vi "Read Tektronix WFM.vi"(8 "Error In":errorcluster, 11 "WFM file Path":path) -> (0 "Error Out":errorcluster, 2 "Waveform out":waveform(dbl), 3 "File out":path)   [LabVIEW 2015]
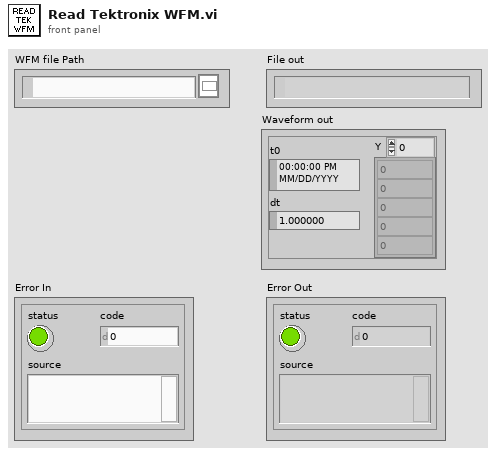
[diagram p1: front panel]
types:
  T1 = typedef "WFM header.ctl" = cluster{"Byte order":u16, "Version":string, "Byte count digits":u8, "Bytes to EOF":i32, "Bytes per point":u8, "Offset of curve buffer":i32, "Label":string, "Number of frames":i32, "Size of header":u16, "Set type":i32, "Number of sets":i32, "Imp dim ref count":i32, "Exp dim ref count":i32, "Data type":i32, "Curve ref count":i32, "Requested FF":i32, "Acquired FF":i32, "Exp dimension 1":T2, "Exp dimension 2":T2, "Imp dimension 1":T3, "Imp dimension 2":T3, "Precharge start offset":i32, "Data start offset":i32, "Postcharge start offset":i32, "Postcharge stop offset":i32, "End of curve buffer offset":i32}
  T2 = typedef "WFM exp dimension.ctl" = cluster{"Scale":dbl, "Offset":dbl, "Size":i32, "Units":string, "Ref point":dbl, "Format":i32, "Storage type":i32, "Trig delay":dbl}
  T3 = typedef "WFM impl dimension.ctl" = cluster{"Scale":dbl, "Offset":dbl, "Size":i32, "Units":string, "Ref point":dbl, "Spacing":i32, "Trig delay":dbl}
  T4 = typedef "WFM file ref.ctl" = cluster{"refnum":refnum<file>, "byte order":enum16{"big-endian, network order", "native, host order", "little-endian"}, "Version":i32}
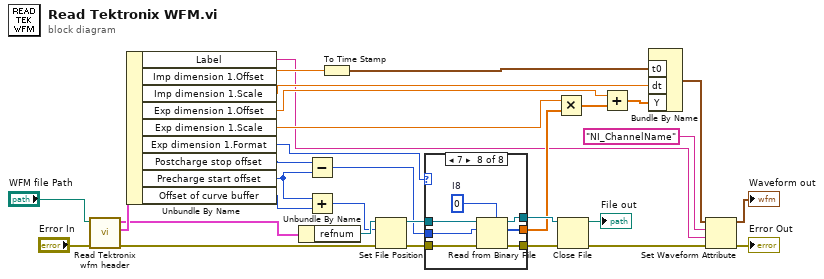
[diagram p0: block diagram]
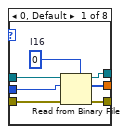
[diagram p2: hidden frame]
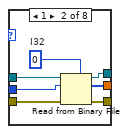
[diagram p3: hidden frame]
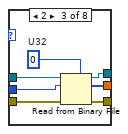
[diagram p4: hidden frame]
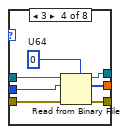
[diagram p5: hidden frame]
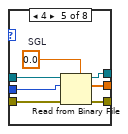
[diagram p6: hidden frame]
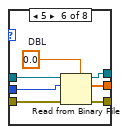
[diagram p7: hidden frame]
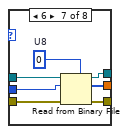
[diagram p8: hidden frame]
diagram:
  n1 = call "Read Tektronix wfm header.vi"("Error In"="Error In", "File Path"="WFM file Path") -> ("Error Out"=w26:errorcluster, "Partial WFM header"=w30:T1, "WFM file ref out"=w29:T4)  [unwired: 7 in]
  n2 = Unbundle By Name(w30) -> ("Label"=w1:string, "Imp dimension 1.Offset"=w18:dbl, "Imp dimension 1.Scale"=w17:dbl, "Exp dimension 1.Offset"=w15:dbl, "Exp dimension 1.Scale"=w14:dbl, "Exp dimension 1.Format"=w12:i32, "Postcharge stop offset"=w11:i32, "Precharge start offset"=w8:i32, "Offset of curve buffer"=w9:i32)
  n3 = Unbundle By Name(w29) -> ("refnum"=w28:refnum<file>)
  n4 = Subtract(x=w11, y=w8) -> (x-y=w10:i32)
  n5 = Add(x=w8, y=w9) -> (x+y=w27:i32)
  n6 = To Time Stamp(1:w18) -> (0:w21:timestamp)
  n7 = Set File Position(offset (in bytes) (0)=w27, refnum=w28, error in=w26) -> (refnum out=w24:refnum<file>, error out=w25:errorcluster)  [unwired: 1 in]
  n8 = case shown="7" w12 {
    tunnel: w25 -> [w38 w45 w52 w59 w66 w73 w80 w87]
    tunnel: w24 -> [w37 w44 w51 w58 w65 w72 w79 w86]
    tunnel: w10 -> [w36 w43 w50 w57 w64 w71 w78 w85]
    tunnel: [w34 w41 w48 w55 w62 w69 w76 w83] -> w23
    tunnel: [w33 w40 w47 w54 w61 w68 w75 w82] -> w22
    tunnel: [w32 w39 w46 w53 w60 w67 w74 w81] -> w13
    frame 0, Default {
      w35 = i16 0  # I16
      n9 = Read from Binary File(5:w35, 8:w38, 10:w36, 11:w37) -> (0:w34:errorcluster, 2:w32:i16[], 3:w33:refnum<file>)  [unwired: 2 in, 1 out]
    }
    frame 1 {
      w42 = 0  # I32
      n10 = Read from Binary File(5:w42, 8:w45, 10:w43, 11:w44) -> (0:w41:errorcluster, 2:w39:i32[], 3:w40:refnum<file>)  [unwired: 2 in, 1 out]
    }
    frame 2 {
      w49 = u32 0  # U32
      n11 = Read from Binary File(5:w49, 8:w52, 10:w50, 11:w51) -> (0:w48:errorcluster, 2:w46:u32[], 3:w47:refnum<file>)  [unwired: 2 in, 1 out]
    }
    frame 3 {
      w56 = u64 0  # U64
      n12 = Read from Binary File(5:w56, 8:w59, 10:w57, 11:w58) -> (0:w55:errorcluster, 2:w53:u64[], 3:w54:refnum<file>)  [unwired: 2 in, 1 out]
    }
    frame 4 {
      w63 = sgl 0.0  # SGL
      n13 = Read from Binary File(5:w63, 8:w66, 10:w64, 11:w65) -> (0:w62:errorcluster, 2:w60:sgl[], 3:w61:refnum<file>)  [unwired: 2 in, 1 out]
    }
    frame 5 {
      w70 = 0.0  # DBL
      n14 = Read from Binary File(5:w70, 8:w73, 10:w71, 11:w72) -> (0:w69:errorcluster, 2:w67:dbl[], 3:w68:refnum<file>)  [unwired: 2 in, 1 out]
    }
    frame 6 {
      w77 = u8 0  # U8
      n15 = Read from Binary File(5:w77, 8:w80, 10:w78, 11:w79) -> (0:w76:errorcluster, 2:w74:u8[], 3:w75:refnum<file>)  [unwired: 2 in, 1 out]
    }
    frame 7 {
      w84 = i8 0  # I8
      n16 = Read from Binary File(5:w84, 8:w87, 10:w85, 11:w86) -> (0:w83:errorcluster, 2:w81:i8[], 3:w82:refnum<file>)  [unwired: 2 in, 1 out]
    }
  }
  n17 = Multiply(x=w14, y=w13) -> (x*y=w16:dbl[])
  n18 = Close File(refnum=w22, error in=w23) -> (path=→"File out":path, error out=w3:errorcluster)
  n19 = Add(x=w15, y=w16) -> (x+y=w20:dbl[])
  n20 = Bundle By Name("t0"=w21, "dt"=w17, "Y"=w20) -> (w6:waveform(dbl))  [unwired: 1 in]
  n21 = Set Waveform Attribute(4:w3, 5:w1, 6:"NI_ChannelName" ("name"), 7:w6) -> (0:→"Error Out":errorcluster, 3:→"Waveform out":waveform(dbl))  [unwired: 1 out]
